vi "loadObjectInfo.vi"(8 "error In":errorcluster, 10 "pathToSTLFiles":path, 11 "Path (dialog)":path) -> (0 "error Out":errorcluster, 2 "availableObjects":T1[](array[typedef]), 3 "objectNames":string[](array[string]))   [LabVIEW 2015]
uses:
  processedObjectInfo.ctl
  objectInfo.ctl
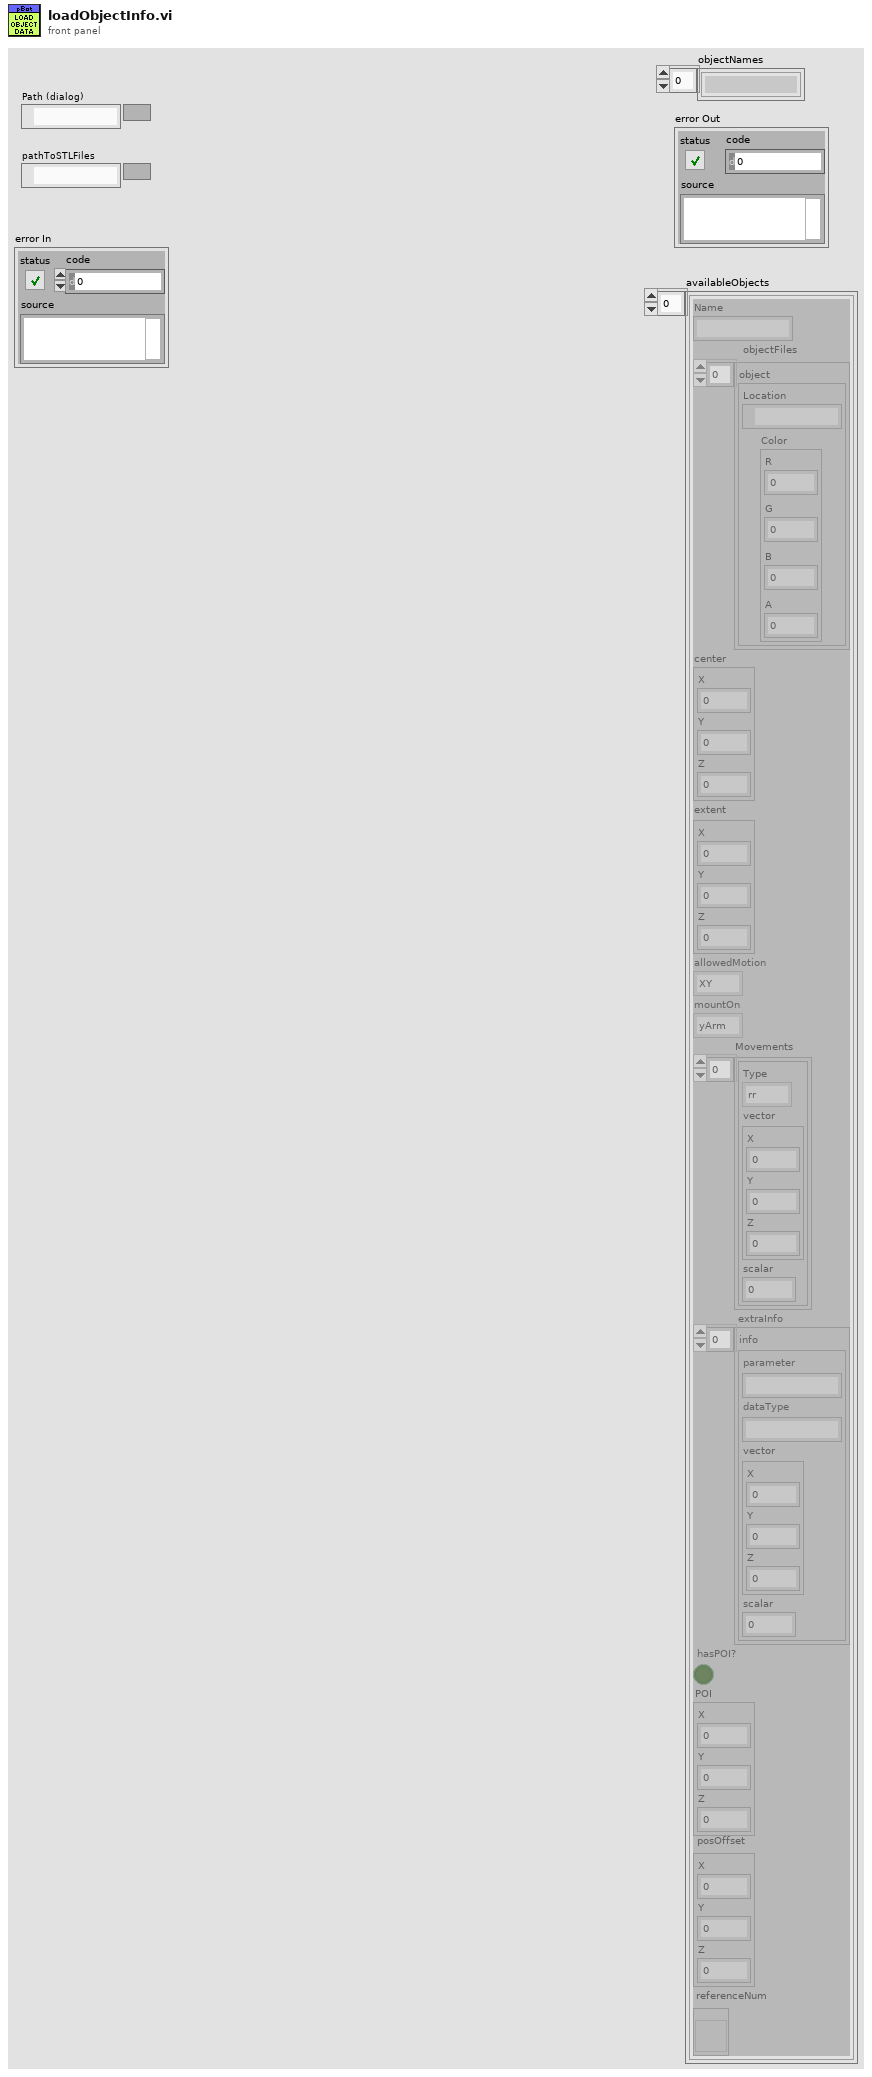
[diagram p1: front panel]
types:
  T1 = typedef "processedObjectInfo.ctl" = cluster{"Name":string, "objectFiles":cluster{"Location":path, "Color":cluster{"R":dbl, "G":dbl, "B":dbl, "A":dbl}}[], "center":cluster{"X":dbl, "Y":dbl, "Z":dbl}, "extent":cluster{"X":dbl, "Y":dbl, "Z":dbl}, "allowedMotion":enum16{"XY", "Z"}, "mountOn":enum16{"yArm", "breadBoard"}, "Movements":cluster{"Type":enum16{"rr", "ra", "tr", "ta"}, "vector":cluster{"X":dbl, "Y":dbl, "Z":dbl}, "scalar":dbl}[], "extraInfo":cluster{"parameter":string, "dataType":string, "vector":cluster{"X":dbl, "Y":dbl, "Z":dbl}, "scalar":dbl}[], "hasPOI?":bool, "POI":cluster{"X":dbl, "Y":dbl, "Z":dbl}, "posOffset":cluster{"X":dbl, "Y":dbl, "Z":dbl}, "referenceNum":refnum<vi>}
  T2 = cluster{"Type":enum16{"rr", "ra", "tr", "ta"}, "vector":cluster{"X":dbl, "Y":dbl, "Z":dbl}, "scalar":dbl}
  T3 = cluster{"Location":path, "Color":cluster{"R":dbl, "G":dbl, "B":dbl, "A":dbl}}
  T4 = typedef "objectInfo.ctl" = cluster{"Name":string, "objectFiles":cluster{"Location":string, "Color":cluster{"R":dbl, "G":dbl, "B":dbl, "A":dbl}}[], "center":cluster{"X":dbl, "Y":dbl, "Z":dbl}, "extent":cluster{"X":dbl, "Y":dbl, "Z":dbl}, "allowedMotion":string, "mountOn":string, "Movements":cluster{"Type":string, "vector":cluster{"X":dbl, "Y":dbl, "Z":dbl}, "scalar":dbl}[], "extraInfo":cluster{"parameter":string, "dataType":string, "vector":cluster{"X":dbl, "Y":dbl, "Z":dbl}, "scalar":dbl}[]}
  T5 = cluster{"Location":string, "Color":cluster{"R":dbl, "G":dbl, "B":dbl, "A":dbl}}[]
  T6 = cluster{"Type":string, "vector":cluster{"X":dbl, "Y":dbl, "Z":dbl}, "scalar":dbl}[]
  T7 = cluster{"parameter":string, "dataType":string, "vector":cluster{"X":dbl, "Y":dbl, "Z":dbl}, "scalar":dbl}[]
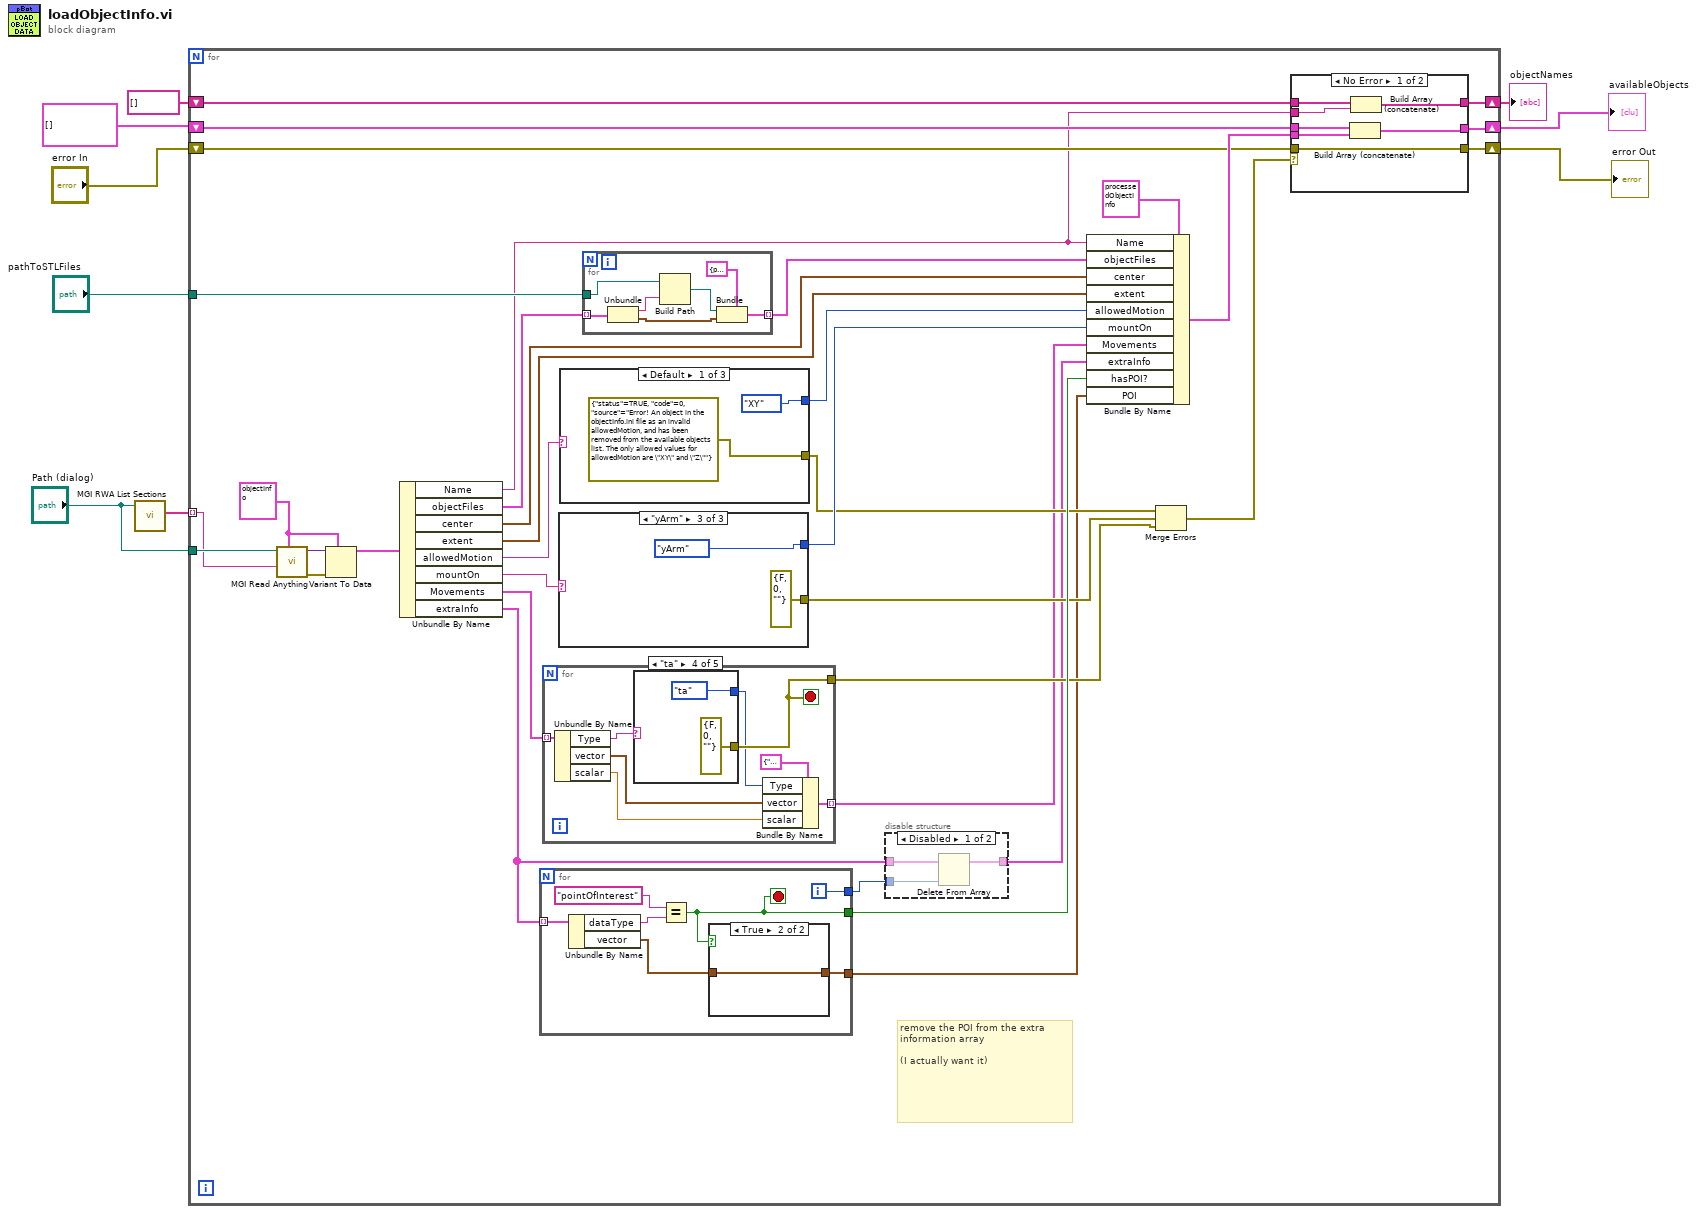
[diagram p0: block diagram]
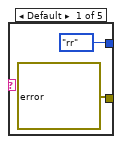
[diagram p3: hidden frame]
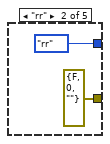
[diagram p4: hidden frame]
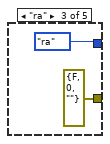
[diagram p5: hidden frame]
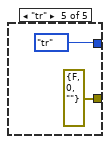
[diagram p6: hidden frame]
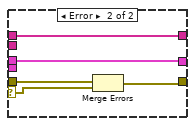
[diagram p7: hidden frame]
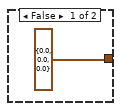
[diagram p8: hidden frame]
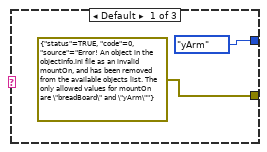
[diagram p9: hidden frame]
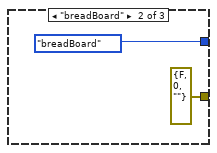
[diagram p10: hidden frame]
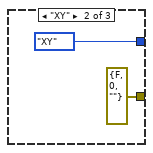
[diagram p11: hidden frame]
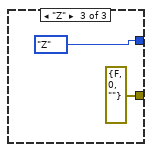
[diagram p12: hidden frame]
diagram:
  n1 = call <userlib>:"MGI RWA List Sections.vi"("Path (dialog)"="Path (dialog)") -> ("Section[]"=w9:string[])  [unwired: 9 in, 1 out]
  n2 = for {
    tunnel: w9 -> [w41] mode=indexing
    tunnel: "Path (dialog)" -> [w42]
    shift-right: [w23] -> w6
    shift-left: T1[] [] ("availableObjects") -> [w24]
    shift-right: [w21] -> w5
    shift-left: "error In" -> [w22]
    tunnel: "pathToSTLFiles" -> [w17]
    shift-right: [w15] -> w1
    shift-left: string[] [] ("availableObjects") -> [w16]
    w40 = T4 {"Name"="", "objectFiles"=[], "center"={"X"=0.0, "Y"=0.0, "Z"=0.0}, "extent"={"X"=0.0, "Y"=0.0, "Z"=0.0}, "allowedMotion"="", "mountOn"="", "Movements"=[], "extraInfo"=[]} ("objectInfo")
    # "remove the POI from the extra information array\n\n(I actually want it)"
    n3 = call <userlib>:"MGI Read Anything.vi"("Type of Anything"=w40, "Section Name (Name of \"Type of Anything\")"=w41, "Path (dialog)"=w42) -> ("Error Out"=w44:errorcluster, "Anything"=w43:variant)  [unwired: 5 in, 2 out]
    n4 = Variant To Data(error in=w44, type=w40, Variant=w43) -> (data=w39:T4)  [unwired: 1 out]
    n5 = Unbundle By Name(w39) -> ("Name"=w14:string, "objectFiles"=w37:T5, "center"=w35:cluster{"X":dbl, "Y":dbl, "Z":dbl}, "extent"=w34:cluster{"X":dbl, "Y":dbl, "Z":dbl}, "allowedMotion"=w33:string, "mountOn"=w31:string, "Movements"=w20:T6, "extraInfo"=w12:T7)
    n6 = for {
      tunnel: w12 -> [w85] mode=indexing
      tunnel: [w82] -> w29
      tunnel: [w80] -> w13
      tunnel: [w79] -> w11
      i -> [w79]
      stop <- w82 stop-if-true
      n7 = Unbundle By Name(w85) -> ("dataType"=w83:string, "vector"=w81:cluster{"X":dbl, "Y":dbl, "Z":dbl})
      n8 = Equal?(x="pointOfInterest" ("y"), y=w83) -> (x = y?=w82:bool)
      n9 = case shown="True" w82 {
        tunnel: w81 -> [_ w87]
        tunnel: [cluster{"X":dbl, "Y":dbl, "Z":dbl} {"X"=0.0, "Y"=0.0, "Z"=0.0} ("POI") w87] -> w80
        frame False {
        }
        frame True {
        }
      }
    }
    n10 = for {
      tunnel: w20 -> [w56] mode=indexing
      tunnel: [w55] -> w19
      tunnel: [w49] -> w18 mode=indexing
      stop <- w55 stop-if-true
      n11 = Unbundle By Name(w56) -> ("Type"=w54:string, "vector"=w51:cluster{"X":dbl, "Y":dbl, "Z":dbl}, "scalar"=w50:dbl)
      n12 = case shown="\"ta\"" w54 {
        tunnel: [enum16{"rr", "ra", "tr", "ta"}."rr" ("Type") enum16{"rr", "ra", "tr", "ta"}."rr" ("Type") enum16{"rr", "ra", "tr", "ta"}."ra" ("Type") enum16{"rr", "ra", "tr", "ta"}."ta" ("Type") enum16{"rr", "ra", "tr", "ta"}."tr" ("Type")] -> w52
        tunnel: [errorcluster {"status"=TRUE, "code"=0, "source"="Error! An object in the objectInfo.ini file as an invalid Movements type, and has been removed from the available objects list. The only allowed values for Movements.Type are \"ta\" (translate absolute), \"tr\" (translate relative), \"ra\" (rotate absolute), and \"rr\" (rotate relative)."} ("error constant") errorcluster {"status"=FALSE, "code"=0, "source"=""} ("error constant") errorcluster {"status"=FALSE, "code"=0, "source"=""} ("error constant") errorcluster {"status"=FALSE, "code"=0, "source"=""} ("error constant") errorcluster {"status"=FALSE, "code"=0, "source"=""} ("error constant")] -> w55
        frame Default {
        }
        frame "rr" {
        }
        frame "ra" {
        }
        frame "ta" {
        }
        frame "tr" {
        }
      }
      n13 = Bundle By Name(cluster=T2 {"Type"=enum."rr", "vector"={"X"=0.0, "Y"=0.0, "Z"=0.0}, "scalar"=0.0} ("Movement"), "Type"=w52, "vector"=w51, "scalar"=w50) -> (w49:T2)
    }
    n14 = case shown="\"yArm\"" w31 {
      tunnel: [enum16{"yArm", "breadBoard"}."yArm" ("mountOn") enum16{"yArm", "breadBoard"}."breadBoard" ("mountOn") enum16{"yArm", "breadBoard"}."yArm" ("mountOn")] -> w30
      tunnel: [errorcluster {"status"=TRUE, "code"=0, "source"="Error! An object in the objectInfo.ini file as an invalid mountOn, and has been removed from the available objects list. The only allowed values for mountOn are \"breadBoard\" and \"yArm\""} ("error constant") errorcluster {"status"=FALSE, "code"=0, "source"=""} ("error constant") errorcluster {"status"=FALSE, "code"=0, "source"=""} ("error constant")] -> w27
      frame Default {
      }
      frame "breadBoard" {
      }
      frame "yArm" {
      }
    }
    n15 = case shown="Default" w33 {
      tunnel: [enum16{"XY", "Z"}."XY" ("allowedMotion") enum16{"XY", "Z"}."XY" ("allowedMotion") enum16{"XY", "Z"}."Z" ("allowedMotion")] -> w32
      tunnel: [errorcluster {"status"=TRUE, "code"=0, "source"="Error! An object in the objectInfo.ini file as an invalid allowedMotion, and has been removed from the available objects list. The only allowed values for allowedMotion are \"XY\" and \"Z\""} ("error constant") errorcluster {"status"=FALSE, "code"=0, "source"=""} ("error constant") errorcluster {"status"=FALSE, "code"=0, "source"=""} ("error constant")] -> w28
      frame Default {
      }
      frame "XY" {
      }
      frame "Z" {
      }
    }
    n16 = for {
      tunnel: w37 -> [w106] mode=indexing
      tunnel: [w103] -> w36 mode=indexing
      tunnel: w17 -> [w102]
      n17 = Unbundle(w106) -> ("Location"=w101:string, "Color"=w104:cluster{"R":dbl, "G":dbl, "B":dbl, "A":dbl})
      n18 = Build Path(base path=w102, name or relative path=w101) -> (appended path=w100:path)
      n19 = Bundle(cluster=T3 {"Location"=path "", "Color"={"R"=0.0, "G"=0.0, "B"=0.0, "A"=0.0}} ("object"), "Location"=w100, "Color"=w104) -> (w103:T3)
    }
    n20 = disable-structure shown="Disabled" {
      disable-tunnel: w12 -> [w47 w48]
      disable-tunnel: w11 -> [w46 _]
      disable-tunnel: [w45 w48] -> w10
      frame Disabled {
        n21 = Delete From Array(array=w47, index=w46) -> (array with subset deleted=w45:T7)  [unwired: 1 in, 1 out]
      }
      frame Enabled {
      }
    }
    n22 = Bundle By Name(cluster=T1 {"Name"="", "objectFiles"=[], "center"={"X"=0.0, "Y"=0.0, "Z"=0.0}, "extent"={"X"=0.0, "Y"=0.0, "Z"=0.0}, "allowedMotion"=enum."XY", "mountOn"=enum."yArm", "Movements"=[], "extraInfo"=[], "hasPOI?"=FALSE, "POI"={"X"=0.0, "Y"=0.0, "Z"=0.0}, "posOffset"={"X"=0.0, "Y"=0.0, "Z"=0.0}, "referenceNum"=refnum} ("processedObjectInfo"), "Name"=w14, "objectFiles"=w36, "center"=w35, "extent"=w34, "allowedMotion"=w32, "mountOn"=w30, "Movements"=w18, "extraInfo"=w10, "hasPOI?"=w29, "POI"=w13) -> (w25:T1)
    n23 = Merge Errors(w28, w27, w19) -> (w26:errorcluster)
    n24 = case shown="No Error" w26 {
      selector: w26 -> [_ w76]
      tunnel: w25 -> [w72 _]
      tunnel: w24 -> [w73 w78]
      tunnel: [w70 w78] -> w23
      tunnel: w22 -> [w71 w77]
      tunnel: [w71 w75] -> w21
      tunnel: w16 -> [w68 w74]
      tunnel: [w69 w74] -> w15
      tunnel: w14 -> [w67 _]
      frame No Error {
        n25 = Build Array (concatenate)(w73, w72) -> (w70:T1[])
        n26 = Build Array (concatenate)(w68, w67) -> (w69:string[])
      }
      frame Error {
        n27 = Merge Errors(w77, w76) -> (w75:errorcluster)
      }
    }
  }
  "availableObjects" <- w6
  "error Out" <- w5
  "objectNames" <- w1
